vi "CodeEncoder.vi"(11 "Code (1-14)":u8) -> (3 "Command":bool[](array[boolean]))   [LabVIEW 2020]
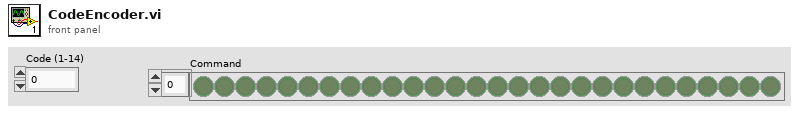
[diagram p1: front panel]
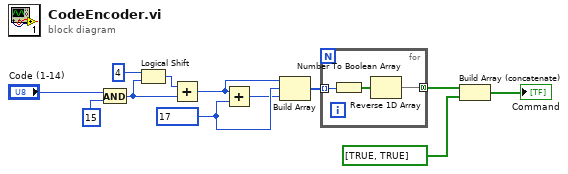
[diagram p0: block diagram]
diagram:
  w4 = u8 17
  n1 = And(x="Code (1-14)", y=u8 15) -> (x .and. y?=w9:u8)
  n2 = Logical Shift(y=i16 4, x=w9) -> (x << y=w10:u8)
  n3 = Add(x=w10, y=w9) -> (x+y=w5:u8)
  n4 = Add(x=w5, y=w4) -> (x+y=w3:u8)
  n5 = Build Array(w5, w4, w3) -> (w2:u8[])
  n6 = for {
    tunnel: w2 -> [w15] mode=indexing
    tunnel: [w13] -> w1 mode=concatenating
    n7 = Number To Boolean Array(number=w15) -> (Boolean array=w14:bool[])
    n8 = Reverse 1D Array(array=w14) -> (reversed array=w13:bool[])
  }
  n9 = Build Array (concatenate)(w1, bool[] [TRUE, TRUE] ("array")) -> (→"Command":bool[])
